vi "FilterBooleanRefs.vi"(8 "error in (no error)":errorcluster, 11 "AllObjs[]":refnum<vi>[](array[refnum])) -> (0 "error out":errorcluster, 3 "AllObjs[] (dup)":refnum<vi>[](array[refnum]))   [LabVIEW 2017, in "NEVSTOP QD Shortcuts.lvlib"]
uses:
  NEVSTOP QD Shortcuts.lvlib
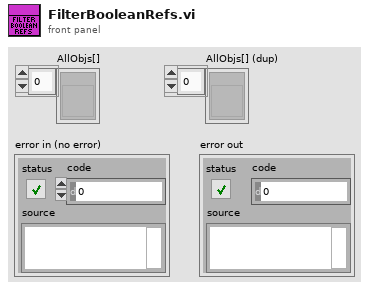
[diagram p1: front panel]
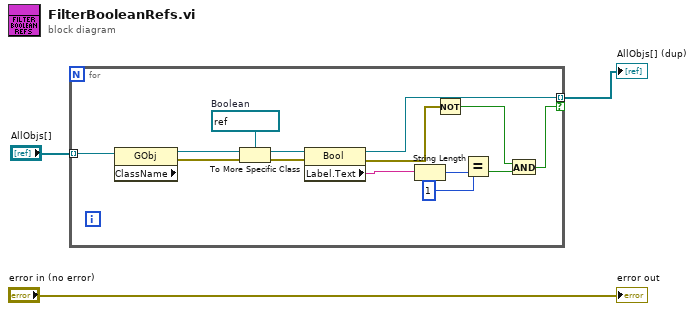
[diagram p0: block diagram]
diagram:
  n1 = for {
    tunnel: "AllObjs[]" -> [w17] mode=indexing
    tunnel: [w12] -> w2 mode=indexing if=w6
    w14 = refnum<vi> refnum  # Boolean
    n2 = property class="GObj" props=["ClassName"](reference=w17) -> (reference out=w16:refnum<vi>, error out=w13:errorcluster)  [unwired: 1 in, 1 out]
    n3 = To More Specific Class(target class=w14, reference=w16, error in=w13) -> (specific class reference=w15:refnum<vi>, error out=w11:errorcluster)
    n4 = property class="Bool"(reference=w15, error in=w11) -> (reference out=w12:refnum<vi>, error out=w10:errorcluster, "Label.Text"=w9:string)
    n5 = String Length(string=w9) -> (length=w8:i32)
    n6 = Not(x=w10) -> (.not. x?=w7:bool)
    n7 = Equal?(x=1, y=w8) -> (x = y?=w5:bool)
    n8 = And(x=w7, y=w5) -> (x .and. y?=w6:bool)
  }
  "AllObjs[] (dup)" <- w2
  "error out" <- "error in (no error)"
